vi "ReadUIEvent.vi"(8 "ErrorIn":errorcluster caption="Error In", 11 "YActor in":refnum<class "YActor.lvclass"> caption="Object In") -> (0 "ErrorOut":errorcluster caption="Error Out", 2 "UIEvent":refnum<user-event>, 3 "YActor out":refnum<class "YActor.lvclass"> caption="Object Out")   [LabVIEW 2021, in "YActor.lvclass"]
uses:
  YActor.lvclass
  YActor.lvclass/YActor.ctl
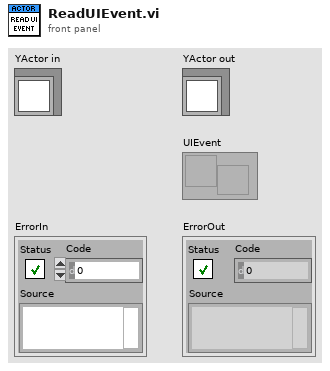
[diagram p1: front panel]
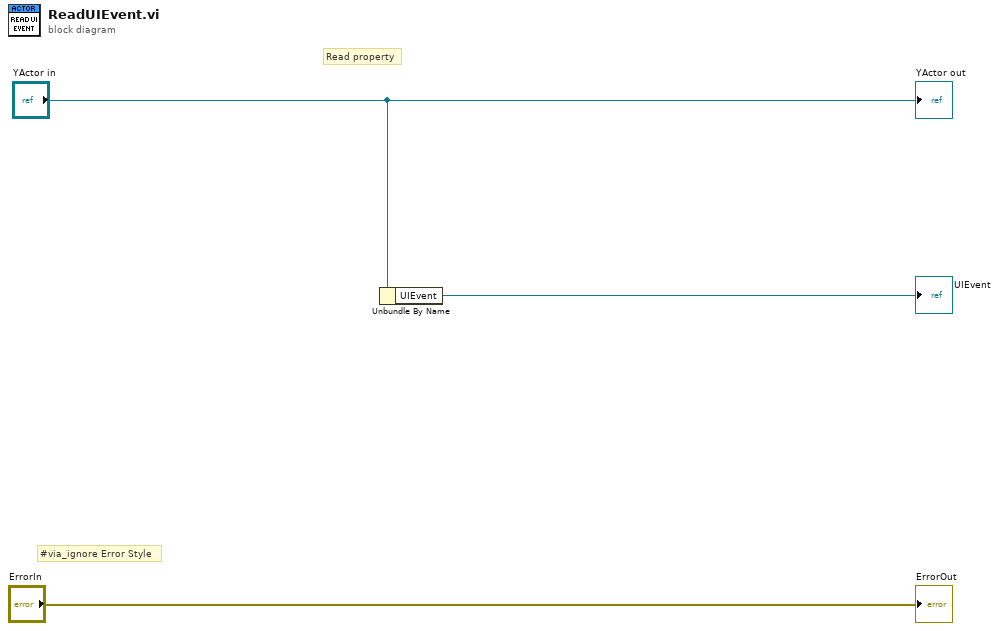
[diagram p0: block diagram]
diagram:
  # "#via_ignore Error Style"
  # "Read property"
  n1 = Unbundle By Name("YActor in") -> ("UIEvent"=→"UIEvent":refnum<user-event>)
  "ErrorOut" <- "ErrorIn"
  "YActor out" <- "YActor in"
